vi "Open Pneumatics V.3.0.vi"   [LabVIEW 2017]
uses:
  <vilib>/Rock Robotics/WPI/Solenoid/WPI_SolenoidChannel.ctl
  <vilib>/Rock Robotics/WPI/Solenoid/WPI_SolenoidOpenSingle.vi
types:
  T1 = typedef "WPI_SolenoidChannel.ctl" = enum8{"Solenoid 0", "Solenoid 1", "Solenoid 2", "Solenoid 3", "Solenoid 4", "Solenoid 5", "Solenoid 6", "Solenoid 7", "Invalid"}
  T2 = typedef "WPI_SolenoidDevRef.ctl" = cluster{"DevStatus":errorcluster, "Pneumatics Control Module":u8, "Forward Solenoid Channel":T1, "Reverse Solenoid Channel":T1}
  T3 = typedef "WPI_CompressorDevRef.ctl" = cluster{"DevStatus":errorcluster, "Pneumatics Control Module":u8}
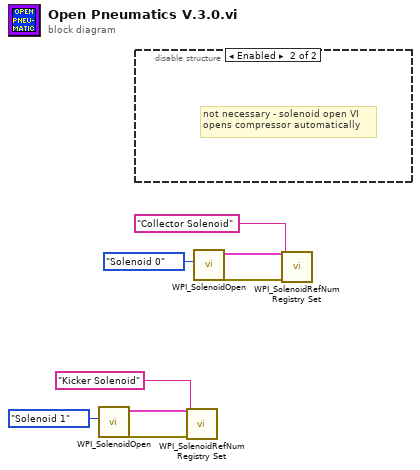
[diagram p0: block diagram]
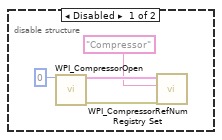
[diagram p2: hidden frame]
diagram:
  n1 = call-poly <vilib>:"WPI_SolenoidOpen.vi"("Solenoid Channel"=WPI_SolenoidChannel."Solenoid 1") -> ("error out"=w1:errorcluster, "SolenoidDevRef"=w3:T2)  [unwired: 9 in]
  n2 = disable-structure shown="Enabled" {
    frame Disabled {
      n3 = call <vilib>:"WPI_CompressorOpen.vi"("Pneumatics Control Module (0)"=u8 0) -> ("CompressorDevRef"=w11:T3, "error out"=w9:errorcluster)  [unwired: 13 in]
      n4 = call <vilib>:"WPI_CompressorRefNum Registry Set.vi"("error in (no error)"=w9, "refnum name"="Compressor", "CompressorDevRef"=w11) -> ()  [unwired: 7 in, 2 out]
    }
    frame Enabled {
      # "not necessary - solenoid open VI\nopens compressor automatically"
    }
  }
  n5 = call <vilib>:"WPI_SolenoidRefNum Registry Set.vi"("error in (no error)"=w1, "refnum name"="Kicker Solenoid", "SolenoidDevRef"=w3) -> ()  [unwired: 7 in, 2 out]
  n6 = call-poly <vilib>:"WPI_SolenoidOpen.vi"("Solenoid Channel"=WPI_SolenoidChannel."Solenoid 0") -> ("error out"=w5:errorcluster, "SolenoidDevRef"=w7:T2)  [unwired: 9 in]
  n7 = call <vilib>:"WPI_SolenoidRefNum Registry Set.vi"("error in (no error)"=w5, "refnum name"="Collector Solenoid", "SolenoidDevRef"=w7) -> ()  [unwired: 7 in, 2 out]
